vi "Write Mouse Event Frame.vi"(10 "Index":i32, 11 "Replay Helper Loop In":T1={"Timeout"=-1, "Run ID"="", "Replay Array Elements"=[], "User Events Metadata"=[]}) -> (3 "Replay Helper Loop Out":T1={"Timeout"=-1, "Run ID"="", "Replay Array Elements"=[], "User Events Metadata"=[]})   [LabVIEW 2026, in "Replay.lvlib"]
uses:
  Replay.lvlib
  Replay Helper Loop.ctl
  User Events Metadata.ctl
  User32.dll
  6371b789-ba5c-4556-852f-409c270b41c6.vi
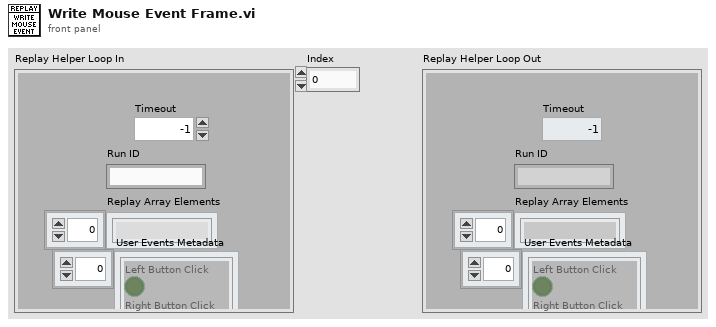
[diagram p1: front panel]
types:
  T1 = typedef "Replay.lvlib/Replay Helper Loop.ctl" = cluster{"Timeout":i32, "Run ID":string, "Replay Array Elements":string[], "User Events Metadata":T2[]}
  T2 = typedef "User Events Metadata.ctl" = cluster{"Cursor Position X":i32, "Cursor Position Y":i32, "Left Button Click":bool, "Right Button Click":bool, "Frame Number":u32}
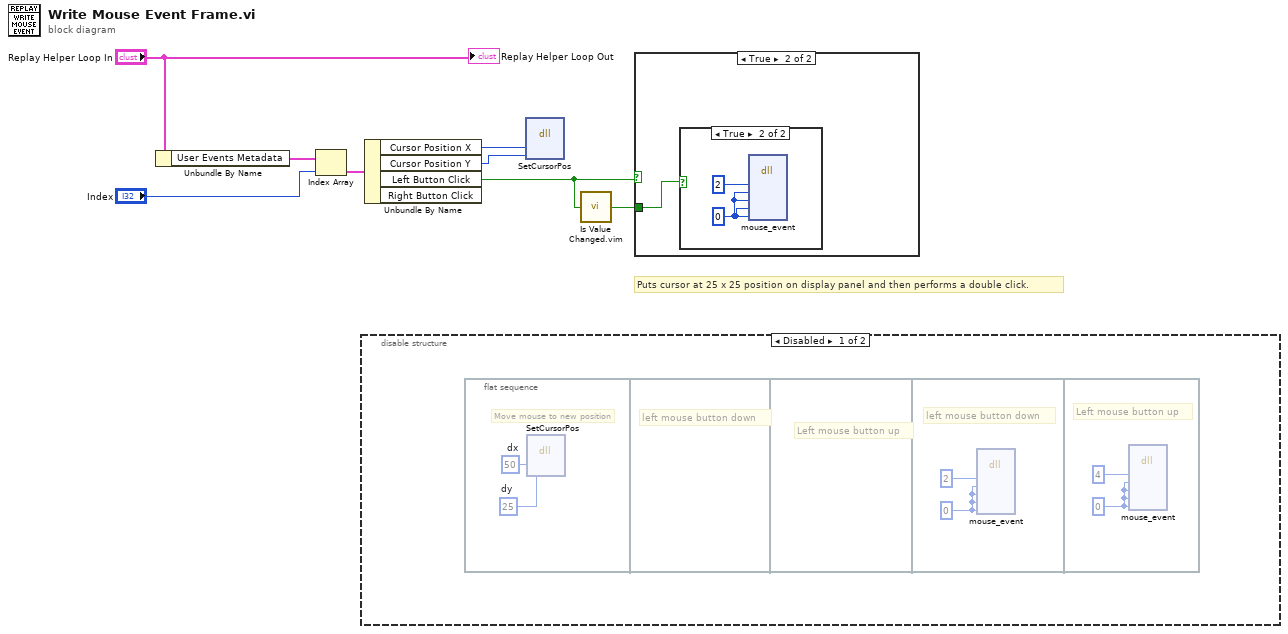
[diagram p0: block diagram]
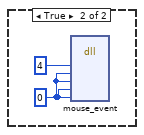
[diagram p4: hidden frame]
diagram:
  # "Puts cursor at 25 x 25 position on display panel and then performs a double click."
  n1 = Unbundle By Name("Replay Helper Loop In") -> ("User Events Metadata"=w7:T2[])
  n2 = Index Array(array=w7, index="Index") -> (element=w5:T2)
  n3 = disable-structure shown="Disabled" {
    frame Disabled {
      n4 = flat-sequence {
        frame #0 {
          w10 = 25  # dy
          w9 = 50  # dx
          # "Move mouse to new position"
          n5 = dll-call lib="User32.dll" fn="SetCursorPos" label="Move mouse to new pos"("dx"=w9, "dy"=w10) -> ()  [unwired: 6 in, 2 out]
        }
        frame #1 {
          # "left mouse button down"
        }
        frame #2 {
          # "Left mouse button up"
        }
        frame #3 {
          w11 = u32 0 ("dy")
          # "left mouse button down"
          n6 = dll-call lib="user32.dll" fn="mouse_event"("dwFlags"=u32 2, "dx"=w11, "dy"=w11, "dwData"=w11, "dwExtraInfo"=w11) -> ()  [unwired: 9 in, 2 out]
        }
        frame #4 {
          w13 = u32 0 ("dy")
          # "Left mouse button up"
          n7 = dll-call lib="user32.dll" fn="mouse_event"("dwFlags"=u32 4, "dx"=w13, "dy"=w13, "dwData"=w13, "dwExtraInfo"=w13) -> ()  [unwired: 9 in, 2 out]
        }
      }
    }
    frame Enabled {
    }
  }
  n8 = Unbundle By Name(w5) -> ("Cursor Position X"=w4:i32, "Cursor Position Y"=w3:i32, "Left Button Click"=w2:bool)  [unwired: 1 out]
  n9 = dll-call lib="User32.dll" fn="SetCursorPos" label="SetCursorPos (User32.dll)"(w4, w3) -> ()  [unwired: 5 in, 3 out]
  n10 = call "Is Value Changed.vim"("value"=w2) -> ("changed or first call?"=w1:bool)
  n11 = case shown="True" w2 {
    tunnel: w1 -> [w15 w18]
    frame False {
      n12 = case shown="False" w15 {
        frame False {
        }
        frame True {
          w16 = u32 0 ("dy")
          n13 = dll-call lib="user32.dll" fn="mouse_event"("dwFlags"=u32 4, "dx"=w16, "dy"=w16, "dwData"=w16, "dwExtraInfo"=w16) -> ()  [unwired: 9 in, 2 out]
        }
      }
    }
    frame True {
      n14 = case shown="True" w18 {
        frame False {
        }
        frame True {
          w19 = u32 0 ("dy")
          n15 = dll-call lib="user32.dll" fn="mouse_event"("dwFlags"=u32 2, "dx"=w19, "dy"=w19, "dwData"=w19, "dwExtraInfo"=w19) -> ()  [unwired: 9 in, 2 out]
        }
      }
    }
  }
  "Replay Helper Loop Out" <- "Replay Helper Loop In"
